vi "VI Tree.vi"   [LabVIEW 2014, in "Agilent ESA PSA Series.lvlib"]
doc: "This is the instrument driver for the Agilent ESA PSA Series. The VI Tree displays all the user-callable VIs of the instrument driver in an organized table."
uses:
  Agilent ESA PSA Series.lvlib
  Configure Trace Operation (Add,Subtract).vi
  Configure Frequency (Center Span).vi
  Configure Trigger Characteristics (RF Burst).vi
  Configure Measurement (Adjacent Channel Power).vi
  Fetch Measurement (Channel Power).vi
  Read Measurement (Channel Power).vi
  Fetch Measurement (Noise Figure).vi
  Configure Range Table (Harmonic Distortion).vi
  Configure Offset And Limits List (Adjacent Channel Power).vi
  Fetch Measurement (Carrier Power - Frequency).vi
  Read Measurement (Carrier Power - Frequency).vi
  Read Measurement (Noise Figure).vi
panel:
  # "(c) 2007-2015 National Instruments.  ALL RIGHTS RESERVED."
  # "SEE DIAGRAM\nFOR VI TREE."
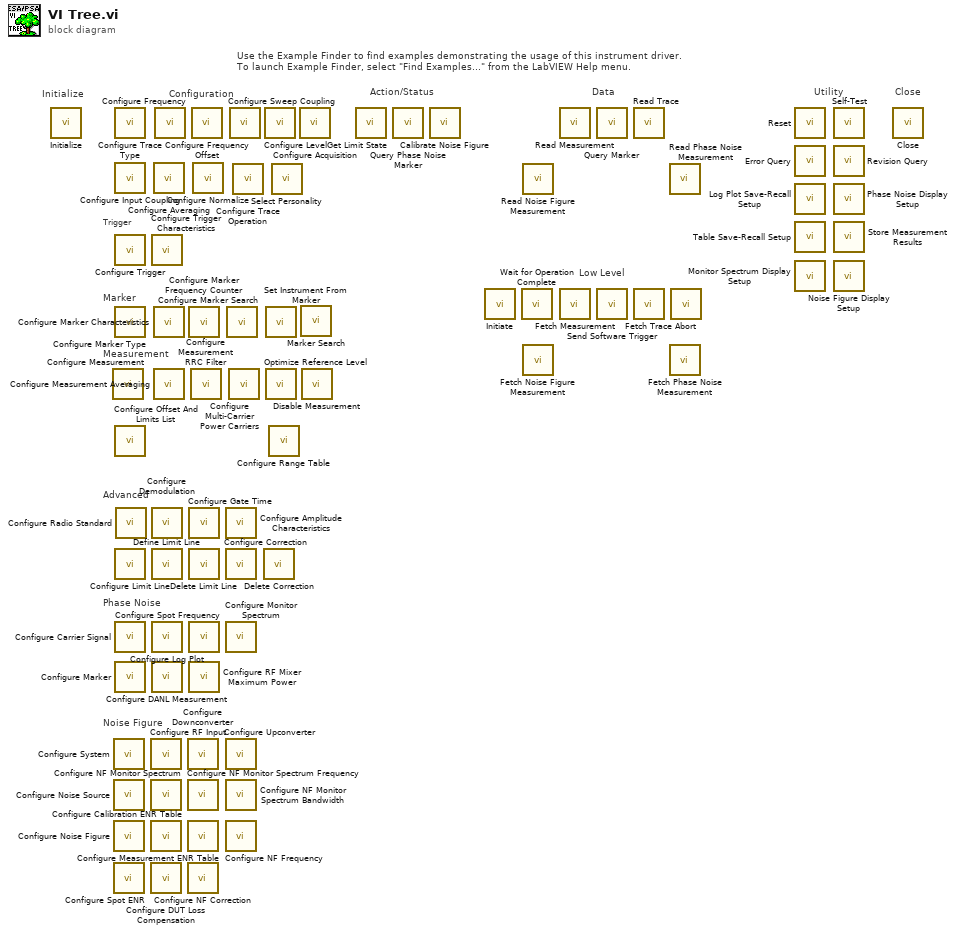
[diagram p0: block diagram]
diagram:
  # "Noise Figure"
  # "Phase Noise"
  # "Trigger"
  # "Marker"
  # "Measurement"
  # "Advanced"
  # "Low Level"
  # "Use the Example Finder to find examples demonstrating the usage of this instrument driver.\nTo launch Example Finder, select \"Find Examples...\" from the LabVIEW Help menu."
  # "Configuration"
  # "Utility"
  # "Data"
  # "Action/Status"
  # "Close"
  # "Initialize"
  n1 = call "Initialize.vi"() -> ()  [unwired: 10 in, 2 out]
  n2 = call-poly "Configure Measurement.vi"() -> ()  [unwired: 14 in, 2 out]
  n3 = call "Configure System.vi"() -> ()  [unwired: 14 in, 2 out]
  n4 = call "Configure Noise Source.vi"() -> ()  [unwired: 10 in, 2 out]
  n5 = call "Configure Noise Figure.vi"() -> ()  [unwired: 14 in, 2 out]
  n6 = call "Configure Spot ENR.vi"() -> ()  [unwired: 14 in, 2 out]
  n7 = call "Configure Trace Type.vi"() -> ()  [unwired: 10 in, 2 out]
  n8 = call "Configure Input Coupling.vi"() -> ()  [unwired: 10 in, 2 out]
  n9 = call "Configure Trigger.vi"() -> ()  [unwired: 14 in, 2 out]
  n10 = call "Configure Marker Type.vi"() -> ()  [unwired: 14 in, 2 out]
  n11 = call-poly "Configure Offset And Limits List.vi"() -> ()  [unwired: 14 in, 2 out]
  n12 = call "Configure Limit Line.vi"() -> ()  [unwired: 14 in, 2 out]
  n13 = call "Configure Carrier Signal.vi"() -> ()  [unwired: 18 in, 2 out]
  n14 = call "Configure Marker.vi"() -> ()  [unwired: 14 in, 2 out]
  n15 = call "Configure Radio Standard.vi"() -> ()  [unwired: 14 in, 2 out]
  n16 = call "Configure RF Input.vi"() -> ()  [unwired: 14 in, 2 out]
  n17 = call "Configure NF Monitor Spectrum.vi"() -> ()  [unwired: 14 in, 2 out]
  n18 = call "Configure Calibration ENR Table.vi"() -> ()  [unwired: 14 in, 2 out]
  n19 = call "Configure DUT Loss Compensation.vi"() -> ()  [unwired: 14 in, 2 out]
  n20 = call-poly "Configure Trigger Characteristics.vi"() -> ()  [unwired: 10 in, 2 out]
  n21 = call "Configure Demodulation.vi"() -> ()  [unwired: 14 in, 2 out]
  n22 = call "Define Limit Line.vi"() -> ()  [unwired: 10 in, 2 out]
  n23 = call "Configure Log Plot.vi"() -> ()  [unwired: 18 in, 2 out]
  n24 = call "Configure DANL Measurement.vi"() -> ()  [unwired: 14 in, 2 out]
  n25 = call "Configure Averaging.vi"() -> ()  [unwired: 10 in, 2 out]
  n26 = call "Configure Marker Characteristics.vi"() -> ()  [unwired: 10 in, 2 out]
  n27 = call "Configure Measurement Averaging.vi"() -> ()  [unwired: 14 in, 2 out]
  n28 = call-poly "Configure Frequency.vi"() -> ()  [unwired: 10 in, 2 out]
  n29 = call "Configure Downconverter.vi"() -> ()  [unwired: 14 in, 2 out]
  n30 = call "Configure NF Monitor Spectrum Frequency.vi"() -> ()  [unwired: 14 in, 2 out]
  n31 = call "Configure Measurement ENR Table.vi"() -> ()  [unwired: 14 in, 2 out]
  n32 = call "Configure NF Correction.vi"() -> ()  [unwired: 14 in, 2 out]
  n33 = call "Configure Marker Frequency Counter.vi"() -> ()  [unwired: 14 in, 2 out]
  n34 = call "Configure Gate Time.vi"() -> ()  [unwired: 14 in, 2 out]
  n35 = call "Delete Limit Line.vi"() -> ()  [unwired: 10 in, 2 out]
  n36 = call "Configure Spot Frequency.vi"() -> ()  [unwired: 18 in, 2 out]
  n37 = call "Configure RF Mixer Maximum Power.vi"() -> ()  [unwired: 14 in, 2 out]
  n38 = call "Configure Measurement RRC Filter.vi"() -> ()  [unwired: 10 in, 2 out]
  n39 = call "Configure Frequency Offset.vi"() -> ()  [unwired: 10 in, 2 out]
  n40 = call "Configure Normalize.vi"() -> ()  [unwired: 10 in, 2 out]
  n41 = call "Configure Amplitude Characteristics.vi"() -> ()  [unwired: 14 in, 2 out]
  n42 = call "Configure Correction.vi"() -> ()  [unwired: 14 in, 2 out]
  n43 = call "Configure Monitor Spectrum.vi"() -> ()  [unwired: 14 in, 2 out]
  n44 = call "Configure Upconverter.vi"() -> ()  [unwired: 14 in, 2 out]
  n45 = call "Configure NF Monitor Spectrum Bandwidth.vi"() -> ()  [unwired: 14 in, 2 out]
  n46 = call "Configure NF Frequency.vi"() -> ()  [unwired: 14 in, 2 out]
  n47 = call "Configure Marker Search.vi"() -> ()  [unwired: 14 in, 2 out]
  n48 = call "Configure Multi-Carrier Power Carriers.vi"() -> ()  [unwired: 14 in, 2 out]
  n49 = call "Configure Sweep Coupling.vi"() -> ()  [unwired: 14 in, 2 out]
  n50 = call-poly "Configure Trace Operation.vi"() -> ()  [unwired: 14 in, 2 out]
  n51 = call "Delete Correction.vi"() -> ()  [unwired: 10 in, 2 out]
  n52 = call "Configure Level.vi"() -> ()  [unwired: 14 in, 2 out]
  n53 = call "Set Instrument From Marker.vi"() -> ()  [unwired: 10 in, 2 out]
  n54 = call "Optimize Reference Level.vi"() -> ()  [unwired: 10 in, 2 out]
  n55 = call-poly "Configure Range Table.vi"() -> ()  [unwired: 14 in, 2 out]
  n56 = call "Select Personality.vi"() -> ()  [unwired: 10 in, 2 out]
  n57 = call "Configure Acquisition.vi"() -> ()  [unwired: 10 in, 2 out]
  n58 = call "Marker Search.vi"() -> ()  [unwired: 10 in, 2 out]
  n59 = call "Disable Measurement.vi"() -> ()  [unwired: 14 in, 2 out]
  n60 = call "Get Limit State.vi"() -> ()  [unwired: 9 in, 3 out]
  n61 = call "Query Phase Noise Marker.vi"() -> ()  [unwired: 12 in, 4 out]
  n62 = call "Calibrate Noise Figure.vi"() -> ()  [unwired: 10 in, 2 out]
  n63 = call "Initiate.vi"() -> ()  [unwired: 10 in, 2 out]
  n64 = call "Wait for Operation Complete.vi"() -> ()  [unwired: 10 in, 2 out]
  n65 = call-poly "Read Noise Figure Measurement.vi"() -> ()  [unwired: 9 in, 3 out]
  n66 = call-poly "Fetch Noise Figure Measurement.vi"() -> ()  [unwired: 9 in, 3 out]
  n67 = call-poly "Read Measurement.vi"() -> ()  [unwired: 8 in, 4 out]
  n68 = call-poly "Fetch Measurement.vi"() -> ()  [unwired: 8 in, 4 out]
  n69 = call "Query Marker.vi"() -> ()  [unwired: 8 in, 4 out]
  n70 = call "Send Software Trigger.vi"() -> ()  [unwired: 10 in, 2 out]
  n71 = call "Read Trace.vi"() -> ()  [unwired: 9 in, 3 out]
  n72 = call "Fetch Trace.vi"() -> ()  [unwired: 7 in, 5 out]
  n73 = call-poly "Read Phase Noise Measurement.vi"() -> ()  [unwired: 8 in, 4 out]
  n74 = call-poly "Fetch Phase Noise Measurement.vi"() -> ()  [unwired: 8 in, 4 out]
  n75 = call "Abort.vi"() -> ()  [unwired: 10 in, 2 out]
  n76 = call "Reset.vi"() -> ()  [unwired: 10 in, 2 out]
  n77 = call "Error Query.vi"() -> ()  [unwired: 8 in, 4 out]
  n78 = call "Log Plot Save-Recall Setup.vi"() -> ()  [unwired: 10 in, 2 out]
  n79 = call "Table Save-Recall Setup.vi"() -> ()  [unwired: 10 in, 2 out]
  n80 = call "Monitor Spectrum Display Setup.vi"() -> ()  [unwired: 14 in, 2 out]
  n81 = call "Self-Test.vi"() -> ()  [unwired: 8 in, 4 out]
  n82 = call "Revision Query.vi"() -> ()  [unwired: 8 in, 4 out]
  n83 = call "Phase Noise Display Setup.vi"() -> ()  [unwired: 10 in, 2 out]
  n84 = call "Store Measurement Results.vi"() -> ()  [unwired: 10 in, 2 out]
  n85 = call "Noise Figure Display Setup.vi"() -> ()  [unwired: 14 in, 2 out]
  n86 = call "Close.vi"() -> ()  [unwired: 11 in, 1 out]
